vi "data manager.vi"(0 "File Type":T1, 1 "action":T3=enum."display", 2 "16Bit Positions":dbl=1000.0, 3 "Z pixels":u32=1024, 5 "# B-lines":u32, 9 "file (use dialog)":path, 11 "error in (no error)":errorcluster, 12 "Save?":bool, 13 "#A-lines per B-line":u32=2048) -> (4 "# elements in queue":i32, 6 "Image":T2(plugin-control), 10 "non empty buffer?":bool, 15 "error out":errorcluster)   [LabVIEW 2018]
uses:
  data manager action.ctl
  type defines/file type.ctl
  Controls/Queue Manager Actions.ctl
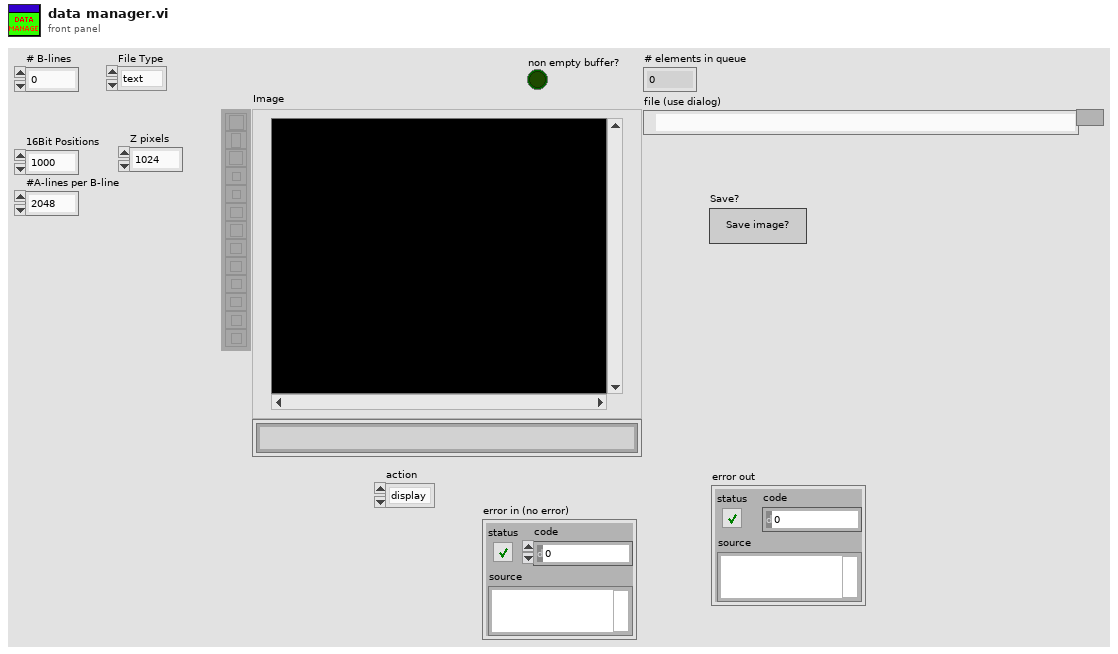
[diagram p1: front panel]
types:
  T1 = typedef "file type.ctl" = enum16{"text", "image", "binary"}
  T2 = typedef "IMAQ Image.ctl" = refnum<image>
  T3 = typedef "data manager action.ctl" = enum16{"Init", "save as text", "Uninit", "open file", "close file", "display", "display and Save"}
  T4 = typedef "Queue Manager Actions.ctl" = enum16{"Init", "Enqueue", "Enqueue All", "Preview Queue", "Dequeue", "Get Status", "Flush Queue", "Flush All Queues", "Release All Queues", "Release Queue", "Enqueue at Opposite End"}
  T5 = typedef "Image Type" = u32
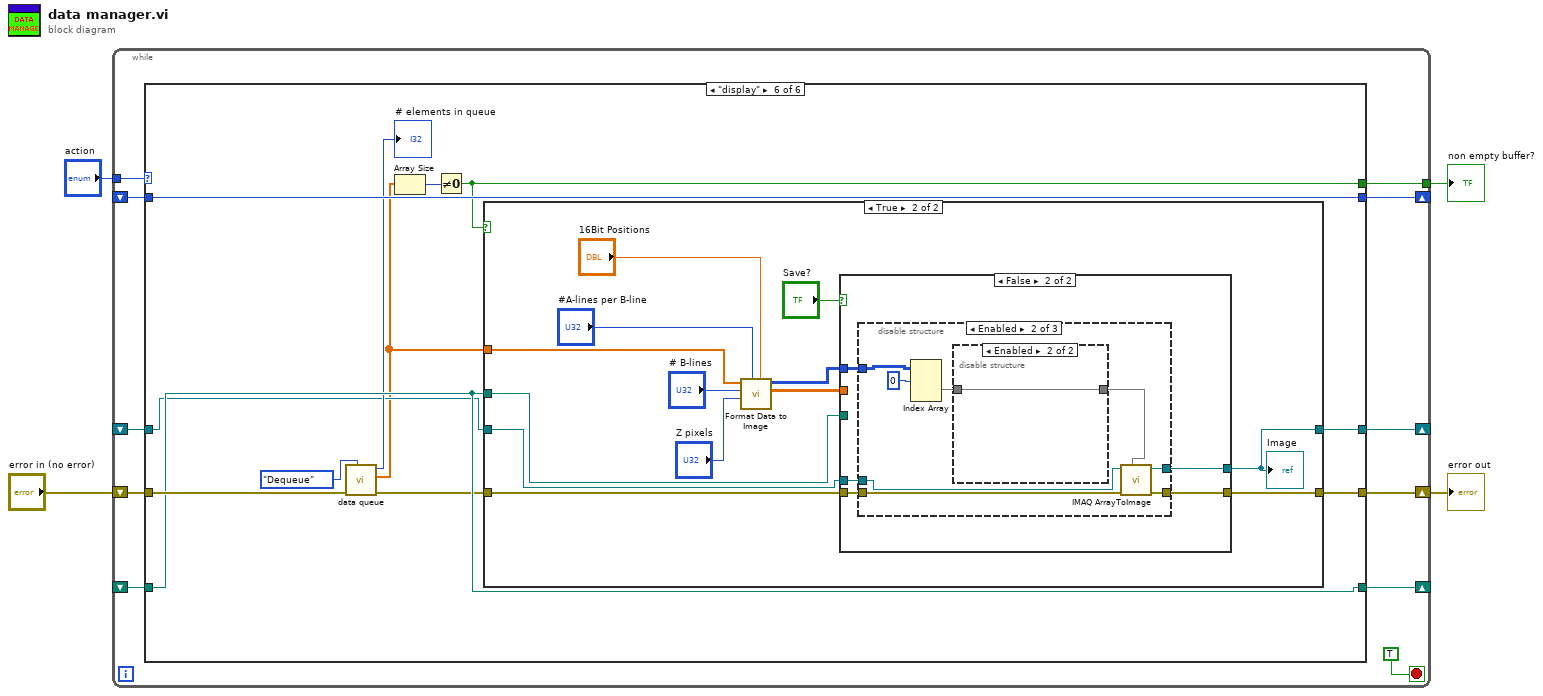
[diagram p0: block diagram]
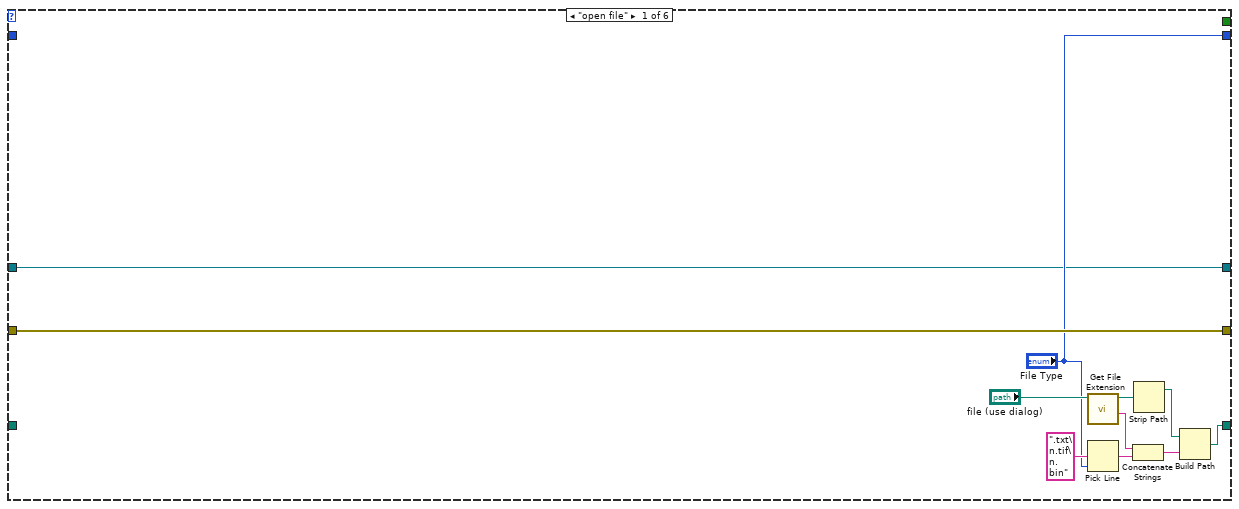
[diagram p2: hidden frame]
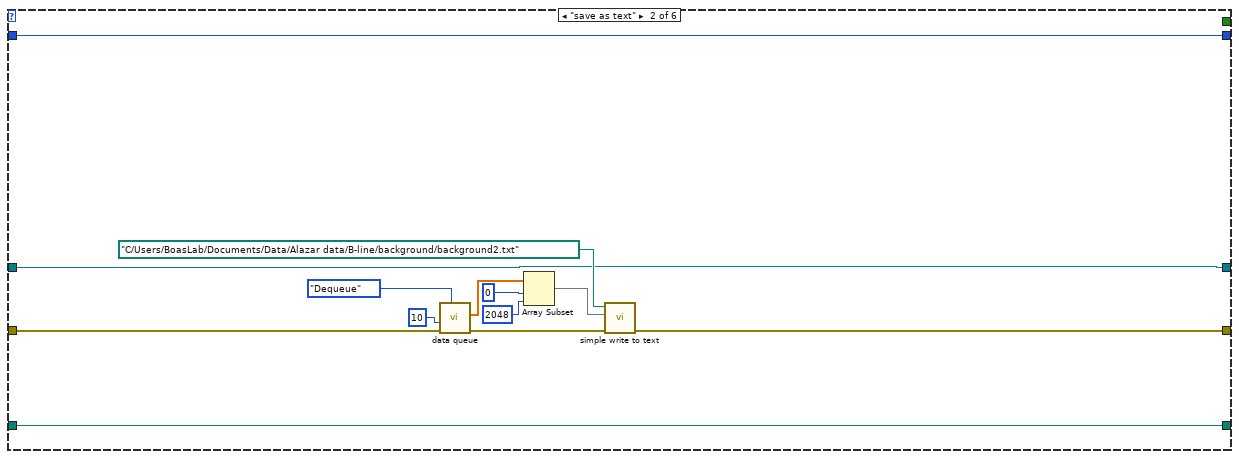
[diagram p3: hidden frame]
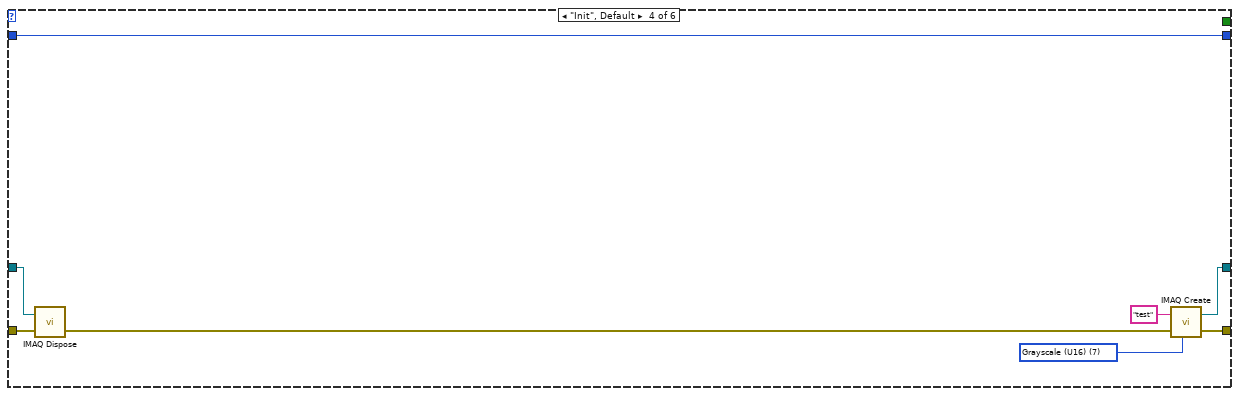
[diagram p5: hidden frame]
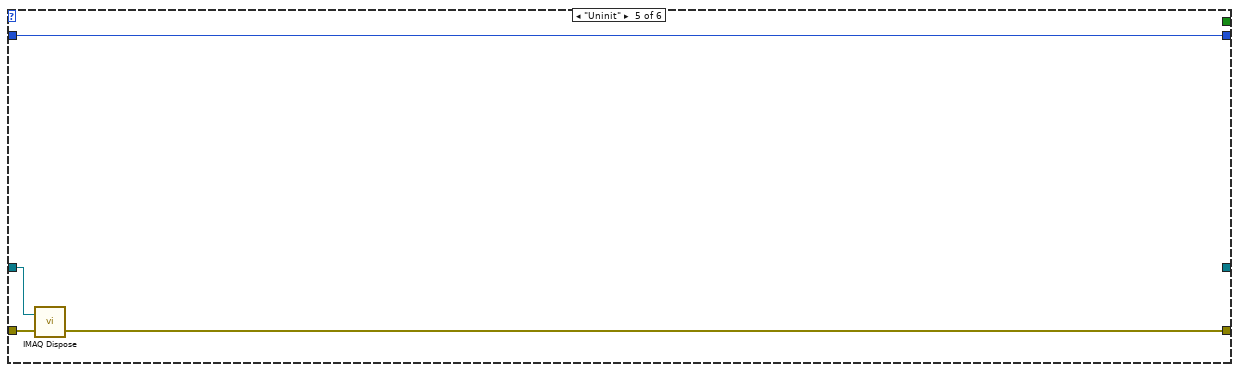
[diagram p6: hidden frame]
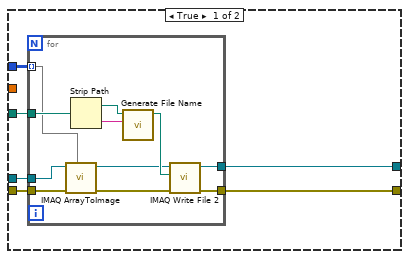
[diagram p8: hidden frame]
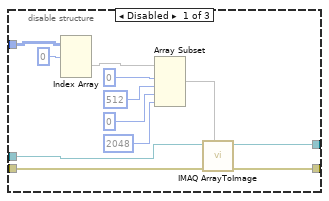
[diagram p9: hidden frame]
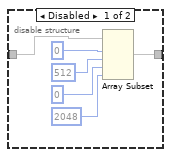
[diagram p10: hidden frame]
diagram:
  n1 = while {
    tunnel: "action" -> [w6]
    shift-right: [w14] -> w3
    shift-left: "error in (no error)" -> [w13]
    shift-right: [w12] -> _
    shift-left: _ -> [w11]
    shift-right: [w10] -> _
    shift-left: _ -> [w9]
    shift-right: [w8] -> _
    shift-left: _ -> [w7]
    tunnel: [w5] -> w1
    stop <- TRUE stop-if-true
    n2 = case shown="\"display\"" w6 {
      tunnel: [w18 w31 w41 w43 w51 w61] -> w14
      tunnel: w13 -> [w18 w39 w41 w47 w53 w64]
      tunnel: [w16 w30 _ w42 _ w62] -> w12
      tunnel: w11 -> [w16 w30 _ w45 w52 w58]
      tunnel: [w22 w29 _ _ _ w60] -> w10
      tunnel: w9 -> [_ w29 _ _ _ w60]
      tunnel: ["File Type" w28 w40 w44 w50 w63] -> w8
      tunnel: w7 -> [_ w28 w40 w44 w50 w63]
      tunnel: [_ _ _ _ _ w55] -> w5
      frame "open file" {
        n3 = call <vilib>:"Get File Extension.vi"("file"="file (use dialog)") -> ("filename without extension"=w19:string, "dup file"=w26:path)  [unwired: 6 in, 3 out]
        n4 = Pick Line(multi-line string=".txt\n.tif\n.bin" ("string"), line index="File Type") -> (output string=w20:string)  [unwired: 1 in]
        n5 = Concatenate Strings(w19, w20) -> (w25:string)
        n6 = Strip Path(path=w26) -> (stripped path=w24:path)  [unwired: 1 out]
        n7 = Build Path(base path=w24, name or relative path=w25) -> (appended path=w22:path)
      }
      frame "save as text" {
        n8 = call "data queue.vi"("Action"=Queue_Manager_Actions."Dequeue", "error in (no error)"=w39, "timeout in ms (-1)"=10) -> ("error out"=w33:errorcluster, "data out"=w37:sgl[])  [unwired: 5 in, 2 out]
        n9 = Array Subset(array=w37, index=0, length=2048) -> (w34:sgl[])
        n10 = call "simple write to text.vi"("error in"=w33, "Background"=w34, "file path (use dialog)"=path "C:/Users/BoasLab/Documents/Data/Alazar data/B-line/background/background2.txt") -> ("error out"=w31:errorcluster)  [unwired: 8 in]
      }
      frame "close file" {
      }
      frame "Init", Default {
        w48 = T5 7 items=["Grayscale (U8)", "Grayscale (I16)", "Grayscale (SGL)", "Complex (CSG)", "RGB (U32)", "HSL (U32)", "RGB (U64)", "Grayscale (U16)"] ("Image Type")
        n11 = call "IMAQ Dispose"("Image"=w45, "error in (no error)"=w47) -> ("error out"=w46:errorcluster)  [unwired: 4 in]
        n12 = call "IMAQ Create"("Image Name"="test", "Image Type"=w48, "error in (no error)"=w46) -> ("New Image"=w42:T2, "error out"=w43:errorcluster)  [unwired: 2 in]
      }
      frame "Uninit" {
        n13 = call "IMAQ Dispose"("Image"=w52, "error in (no error)"=w53) -> ("error out"=w51:errorcluster)  [unwired: 4 in]
      }
      frame "display" {
        n14 = call "data queue.vi"("Action"=Queue_Manager_Actions."Dequeue", "error in (no error)"=w64) -> ("error out"=w54:errorcluster, "data out"=w57:sgl[], "# elements in queue"=→"# elements in queue":i32)  [unwired: 6 in, 1 out]
        n15 = Array Size(array=w57) -> (size(s)=w56:i32)
        n16 = Not Equal To 0?(x=w56) -> (x != 0?=w55:bool)
        n17 = case shown="True" w55 {
          tunnel: w57 -> [_ w80]
          tunnel: [w66 w79] -> w62
          tunnel: [w67 w78] -> w61
          tunnel: w60 -> [_ w76]
          tunnel: w58 -> [w66 w75]
          tunnel: w54 -> [w67 w72]
          frame False {
          }
          frame True {
            n18 = call "Format Data to Image.vi"("16Bit Positions"="16Bit Positions", "#A-lines per B-line"="#A-lines per B-line", "Z pixels"="Z pixels", "# B-lines"="# B-lines", "data in"=w80) -> ("float data"=w71:sgl[][][], "U16bit data"=w74:u16[][][])  [unwired: 5 in]
            n19 = case shown="False" "Save?" {
              tunnel: [w86 w102] -> w79
              tunnel: [w82 w101] -> w78
              tunnel: w76 -> [w85 _]
              tunnel: w75 -> [w84 w100]
              tunnel: w74 -> [w81 w98]
              tunnel: w72 -> [w83 w99]
              tunnel: w71 -> [_ _]
              frame True {
                n20 = for {
                  tunnel: [w97] -> w86
                  tunnel: w85 -> [w96]
                  tunnel: w84 -> [w93]
                  tunnel: w81 -> [w87] mode=indexing
                  tunnel: w83 -> [w89]
                  tunnel: [w88] -> w82
                  n21 = call "IMAQ ArrayToImage"("Image Pixels (U16)"=w87, "error in (no error)"=w89, "Image"=w93) -> ("error out"=w92:errorcluster, "Image Out"=w91:T2)  [unwired: 7 in]
                  n22 = Strip Path(path=w96) -> (stripped path=w90:path, name=w95:string)
                  n23 = call "Generate File Name.vi"("name or relative path"=w95, "base path"=w90) -> ("appended path"=w94:path)  [unwired: 9 in]
                  n24 = call-poly "IMAQ Write File 2"("error in (no error)"=w92, "File Path"=w94, "Image"=w91) -> ("error out"=w88:errorcluster, "Image Out (duplicate)"=w97:T2)  [unwired: 7 in]
                }
              }
              frame False {
                n25 = disable-structure shown="Enabled" {
                  disable-tunnel: [w114 w122 _] -> w102
                  disable-tunnel: [w113 w121 _] -> w101
                  disable-tunnel: w100 -> [w112 w120 _]
                  disable-tunnel: w98 -> [w111 w116 _]
                  disable-tunnel: w99 -> [w109 w118 _]
                  frame Disabled {
                    n26 = Index Array(array=w111, index (dim 0)=0 ("index (page)")) -> (element=w108:u16[][])  [unwired: 2 in]
                    n27 = Array Subset(array=w108, index (row)=0 ("index"), length (row)=512 ("length"), index (col)=0 ("index"), length (col)=2048 ("length")) -> (w103:u16[][])
                    n28 = call "IMAQ ArrayToImage"("Image Pixels (U16)"=w103, "error in (no error)"=w109, "Image"=w112) -> ("error out"=w113:errorcluster, "Image Out"=w114:T2)  [unwired: 7 in]
                  }
                  frame Enabled {
                    n29 = Index Array(array=w116, index (dim 0)=0 ("index (page)")) -> (element=w117:u16[][])  [unwired: 2 in]
                    n30 = disable-structure shown="Enabled" {
                      disable-tunnel: w117 -> [w128 w129]
                      disable-tunnel: [w123 w129] -> w115
                      frame Disabled {
                        n31 = Array Subset(array=w128, index (row)=0 ("index"), length (row)=512 ("length"), index (col)=0 ("index"), length (col)=2048 ("length")) -> (w123:u16[][])
                      }
                      frame Enabled {
                      }
                    }
                    n32 = call "IMAQ ArrayToImage"("Image Pixels (U16)"=w115, "error in (no error)"=w118, "Image"=w120) -> ("error out"=w121:errorcluster, "Image Out"=w122:T2)  [unwired: 7 in]
                  }
                  frame Disabled {
                  }
                }
              }
            }
            "Image" <- w79
          }
        }
      }
    }
  }
  "error out" <- w3
  "non empty buffer?" <- w1
